vi "Initialize Frame.vi"(8 "Error In":errorcluster, 10 "Size":T1, 11 "Display Manager In":refnum<class "Display Manager.lvclass">) -> (0 "Error Out":errorcluster, 3 "Display Manager Out":refnum<class "Display Manager.lvclass">)   [LabVIEW 2021, in "Display Manager.lvclass"]
uses:
  Display Manager.lvclass
  Display Utilities/Public/Controls/2D Dimensions.ctl
  Accessors/Size/Set Size.vi
  Accessors/Frame/Set Frame.vi
  Display Utilities/Display Utilities.lvlib
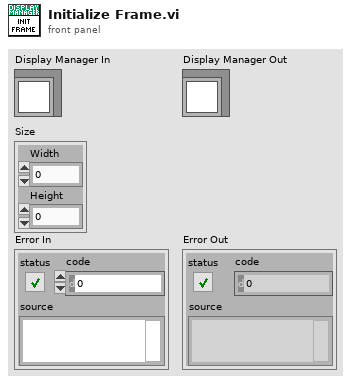
[diagram p1: front panel]
types:
  T1 = typedef "Display Utilities.lvlib/2D Dimensions.ctl" = cluster{"Width":i32, "Height":i32}
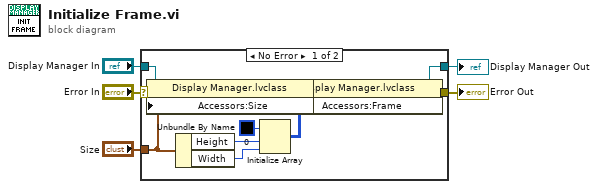
[diagram p0: block diagram]
diagram:
  n1 = case shown="No Error" "Error In" {
    selector: "Error In" -> [w16 w17]
    tunnel: "Display Manager In" -> [w15 w18]
    tunnel: [w6 w18] -> w3
    tunnel: [w14 w17] -> w2
    tunnel: "Size" -> [w12 _]
    frame No Error {
      n2 = property class="Display Manager.lvclass"(reference=w15, error in=w16, "Accessors:Size"=w12) -> (reference out=w7:refnum<class "Display Manager.lvclass">, error out=w8:errorcluster)
      n3 = Unbundle By Name(w12) -> ("Height"=w11:i32, "Width"=w10:i32)
      n4 = Initialize Array(u32 0 ("Color"), w11, w10) -> (w9:u32[][])
      n5 = property class="Display Manager.lvclass"(reference=w7, error in=w8, "Accessors:Frame"=w9) -> (reference out=w6:refnum<class "Display Manager.lvclass">, error out=w14:errorcluster)
    }
    frame Error {
    }
  }
  "Display Manager Out" <- w3
  "Error Out" <- w2
